vi "autoshutdown_ITC.vi"   [LabVIEW 2016]
uses:
  CryoTUM-V1.0/Instrument_Setup.vi
types:
  T1 = typedef "ITCIO.ctl" = cluster{"Address":T2, "Version":T3, "Ch 1 dec places":i16, "Ch 2 dec places":i16, "Ch 3 dec places":i16, "Ch1 Name":string, "Ch2 Name":string, "Ch3 Name":string}
  T2 = typedef "OxfordAddress.ctl" = cluster{"Com Port":i32, "ISOBUS Address":i32, "GPIB Address":i16, "Communication":enum16{"RS232", "ISOBUS", "GPIB", "Gateway"}}
  T3 = typedef "ITCVersion.ctl" = enum16{"ITC502", "ITC503", "ITC601"}
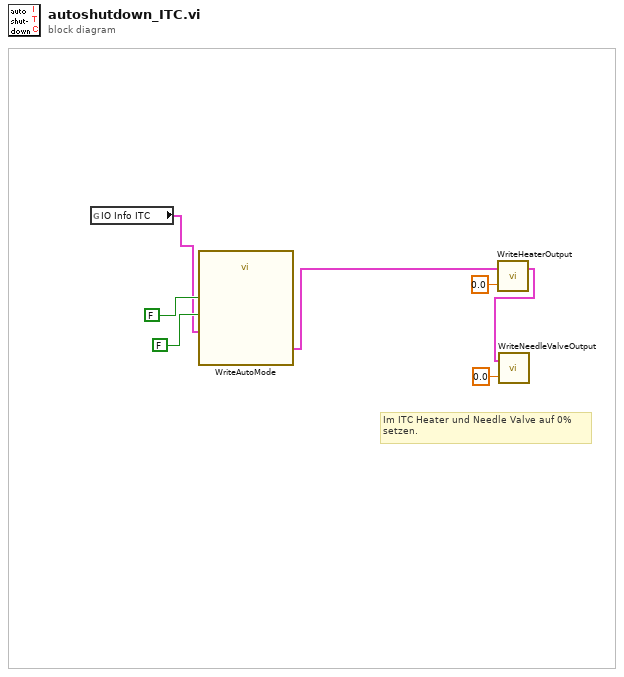
[diagram p0: block diagram]
diagram:
  # "Im ITC Heater und Needle Valve auf 0%\nsetzen."
  n1 = global read "Instrument_Setup.vi" "IO Info ITC"() -> (w1:T1)
  n2 = call "WriteAutoMode.vi"("Auto Needle Valve"=FALSE, "Auto Heat"=FALSE, "ITC IO Info"=w1) -> ("ITC IO Info"=w2:T1)
  n3 = call "WriteHeaterOutput.vi"("Heater Output (%)"=0.0, "ITC IO Info"=w2) -> ("ITC IO Info"=w5:T1)  [unwired: 1 in]
  n4 = call "WriteNeedleValveOutput.vi"("Needle Valve Output (%"=0.0, "ITC IO Info"=w5) -> ()  [unwired: 1 in, 1 out]
